vi "Occurence.vi"() -> ()   [LabVIEW 2020]
panel:
  out "Numbers 2":i32
  out "Numbers":i32
  in  "Start":bool
  in  "stop":bool
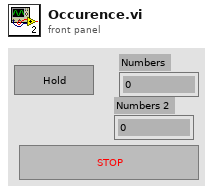
[diagram p1: front panel]
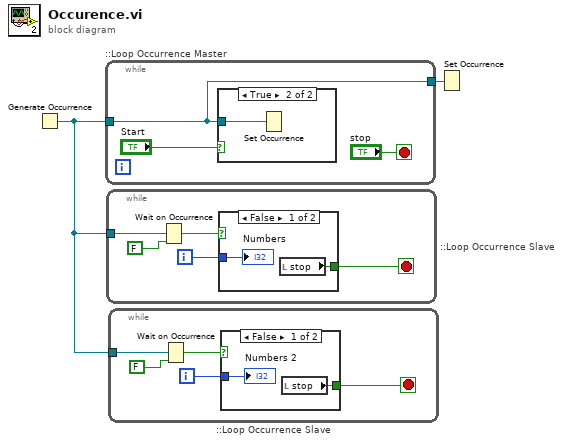
[diagram p0: block diagram]
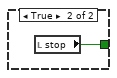
[diagram p2: hidden frame]
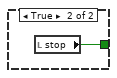
[diagram p3: hidden frame]
diagram:
  n1 = Generate Occurrence() -> (w1:refnum<k4>)
  n2 = while "::Loop Occurrence Master" {
    tunnel: w1 -> [w3]
    tunnel: [w3] -> w2
    stop <- "stop" stop-if-true
    n3 = case shown="True" "Start" {
      tunnel: w3 -> [_ w6]
      frame False {
      }
      frame True {
        n4 = Set Occurrence(w6) -> ()
      }
    }
  }
  n5 = while "::Loop Occurrence Slave" {
    tunnel: w1 -> [w11]
    i -> [w8]
    stop <- w7 stop-if-true
    n6 = Wait on Occurrence(1:FALSE ("ignore previous (T)"), 2:w11) -> (0:w9:bool)  [unwired: 1 in]
    n7 = case shown="False" w9 {
      tunnel: w8 -> [w13 _]
      tunnel: [w12 w14] -> w7
      frame False {
        n8 = local read "stop"() -> (w12:bool)
        "Numbers" <- w13
      }
      frame True {
        n9 = local read "stop"() -> (w14:bool)
      }
    }
  }
  n10 = while "::Loop Occurrence Slave" {
    tunnel: w1 -> [w19]
    i -> [w16]
    stop <- w15 stop-if-true
    n11 = Wait on Occurrence(1:FALSE ("ignore previous (T)"), 2:w19) -> (0:w17:bool)  [unwired: 1 in]
    n12 = case shown="False" w17 {
      tunnel: w16 -> [w21 _]
      tunnel: [w20 w22] -> w15
      frame False {
        n13 = local read "stop"() -> (w20:bool)
        "Numbers 2" <- w21
      }
      frame True {
        n14 = local read "stop"() -> (w22:bool)
      }
    }
  }
  n15 = Set Occurrence(w2) -> ()
